vi "INST_MODE.vi"(0 "Session In":refnum<visa-resource-name>="TCPIP0::K-N90X0A-00005.local::inst0::INSTR", 2 "RO(T)":bool, 11 "error in":errorcluster {"code" format="%.0x"}, 12 "MODE":T1(ring), 13 "Timeout":u32=3000) -> (3 "mode":string, 4 "Session Out":refnum<visa-resource-name>, 15 "error out":errorcluster {"code" format="%.0x"})   [LabVIEW 2018]
doc: "Set the MODE of the 9010\n0: SA\n1: GSM\n2: LTE FDD\n3: LTE TDD"
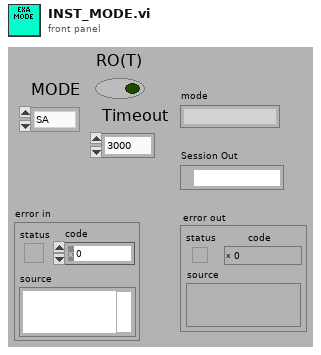
[diagram p1: front panel]
types:
  T1 = enum16{"SA", "EDGE/GSM", "LTE TDD", "LTE FDD", "PNOISE"}
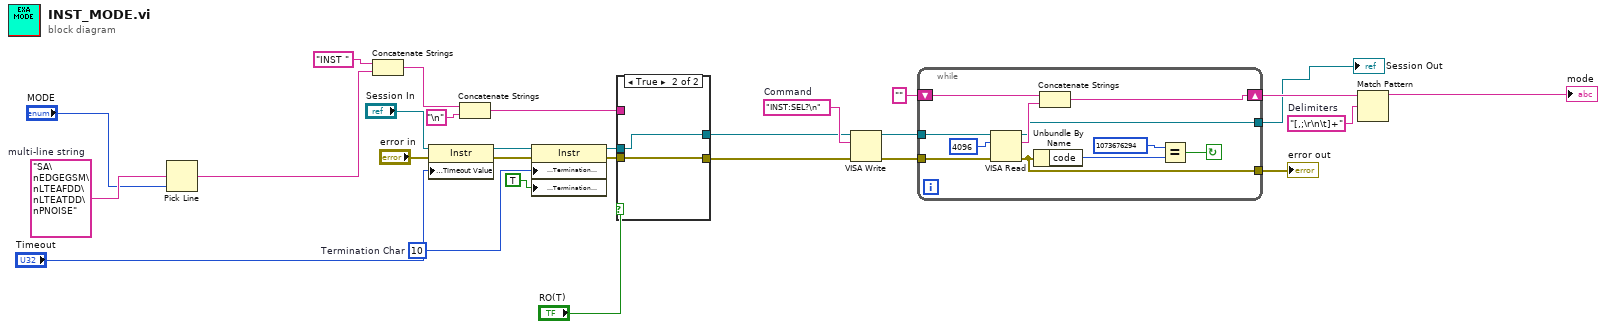
[diagram p0: block diagram]
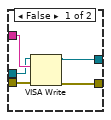
[diagram p2: hidden frame]
diagram:
  w3 = "SA\nEDGEGSM\nLTEAFDD\nLTEATDD\nPNOISE"  # multi-line string
  w9 = "[,;\r\n\t]+"  # Delimiters
  w11 = "INST:SEL?\n"  # Command
  w23 = u8 10  # Termination Char
  n1 = Pick Line(multi-line string=w3, line index="MODE") -> (output string=w4:string)  [unwired: 1 in]
  n2 = Concatenate Strings("INST " ("staticText"), w4) -> (w17:string)
  n3 = property class="Instr"(reference="Session In", error in="error in", "General Settings:Timeout Value"="Timeout") -> (reference out=w22:refnum<visa-resource-name>, error out=w25:errorcluster)
  n4 = Concatenate Strings(w17, "\n" ("StaticText")) -> (w18:string)
  n5 = property class="Instr"(reference=w22, error in=w25, "Message Based Settings:Termination Character"=w23, "Message Based Settings:Termination Character Enable"=TRUE ("enable")) -> (reference out=w7:refnum<visa-resource-name>, error out=w24:errorcluster)
  n6 = case shown="True" "RO(T)" {
    tunnel: w24 -> [w33 w34]
    tunnel: [w32 w34] -> w19
    tunnel: w18 -> [w31 _]
    tunnel: w7 -> [w30 w35]
    tunnel: [w29 w35] -> w6
    frame False {
      n7 = VISA Write(VISA resource name=w30, write buffer=w31, error in (no error)=w33) -> (VISA resource name out=w29:refnum<visa-resource-name>, error out=w32:errorcluster)  [unwired: 1 out]
    }
    frame True {
    }
  }
  n8 = VISA Write(VISA resource name=w6, write buffer=w11, error in (no error)=w19) -> (VISA resource name out=w15:refnum<visa-resource-name>, error out=w14:errorcluster)  [unwired: 1 out]
  n9 = while {
    tunnel: w15 -> [w43]
    shift-right: [w37] -> w8
    shift-left: "" -> [w42]
    tunnel: w14 -> [w40]
    tunnel: [w39] -> w13
    tunnel: [w36] -> w5
    stop <- w38 continue-if-true
    n10 = VISA Read(VISA resource name=w43, byte count=u32 4096 ("byte count (0)"), error in (no error)=w40) -> (VISA resource name out=w36:refnum<visa-resource-name>, read buffer=w41:string, error out=w39:errorcluster)  [unwired: 1 out]
    n11 = Unbundle By Name(w39) -> ("code"=w45:i32)
    n12 = Concatenate Strings(w42, w41) -> (w37:string)
    n13 = Equal?(x=1073676294, y=w45) -> (x = y?=w38:bool)
  }
  "error out" <- w13
  "Session Out" <- w5
  n14 = Match Pattern(string=w8, regular expression=w9) -> (before substring=→"mode":string)  [unwired: 4 out]
